vi "Generate Incremental Array.vi"(1 "Array Size":i32, 2 "Starting Element":dbl) -> (0 "Output Array":dbl[](array[numeric]))   [LabVIEW 2017]
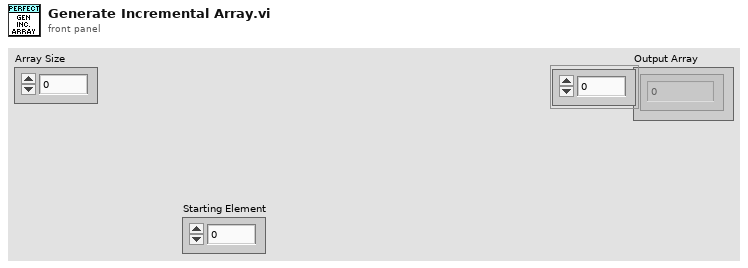
[diagram p1: front panel]
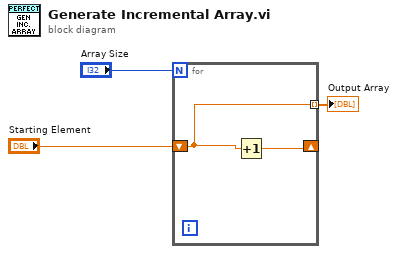
[diagram p0: block diagram]
diagram:
  n1 = for {
    N: "Array Size" -> [_]
    shift-right: [w4] -> _
    shift-left: "Starting Element" -> [w5]
    tunnel: [w5] -> w1 mode=indexing
    n2 = Increment(x=w5) -> (x+1=w4:dbl)
  }
  "Output Array" <- w1
